vi "Simple Test 1.vi"() -> ()   [LabVIEW 2014]
uses:
  <vilib>/Aledyne-TSXperts/Arduino Compatible Compiler for LabVIEW/addons/Arduino MPU60X0/Arduino MPU60X0.lvlib
panel:
  out "A out":dbl
  in  "A":dbl
  out "Error Out":errorcluster
  in  "Error In":errorcluster
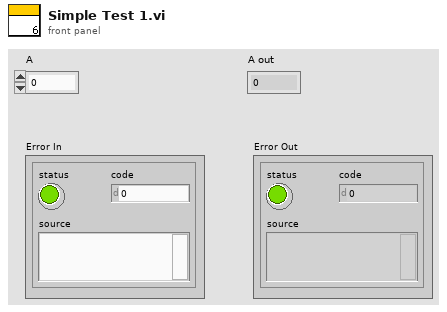
[diagram p1: front panel]
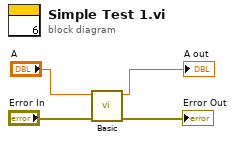
[diagram p0: block diagram]
diagram:
  n1 = call <vilib>:"Basic.vi"("Error In"="Error In", "A"="A") -> ("Error Out"=→"Error Out":errorcluster, "A out"=→"A out":dbl)  [unwired: 8 in]
